vi "platform2Channel.vi"(11 "Array":dbl[](array[numeric])) -> (3 "DAQmx Channel":string)   [LabVIEW 2017]
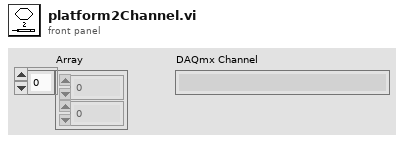
[diagram p1: front panel]
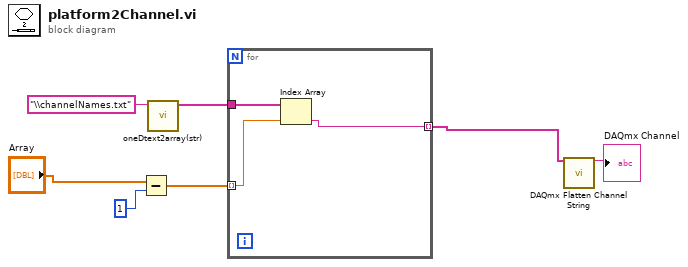
[diagram p0: block diagram]
diagram:
  n1 = Subtract(x="Array", y=1) -> (x-y=w3:dbl[])
  n2 = call "oneDtext2array(str).vi"("String"="\\channelNames.txt") -> ("text"=w6:string[])  [unwired: 10 in]
  n3 = for {
    tunnel: w6 -> [w10]
    tunnel: w3 -> [w9] mode=indexing
    tunnel: [w8] -> w2 mode=indexing
    n4 = Index Array(array=w10, index=w9) -> (element=w8:string)
  }
  n5 = call <vilib>:"DAQmx Flatten Channel String.vi"("names in"=w2) -> ("names out"=→"DAQmx Channel":string)  [unwired: 13 in, 1 out]
